vi "CalibrationPathConstants.vi"() -> (0 "PSU3 TachPath":T1=path "Z:/Data/Calibration/Tachometer/PSU3_TachCalibration.csv", 1 "PSU2 RevTachPath":T1=path "Z:/Data/Calibration/Reverse Tachometer/PSU2_RevTachCalibration.csv", 2 "PSU2 TachPath":T1=path "Z:/Data/Calibration/Tachometer/PSU2_TachCalibration.csv", 3 "CryoPath":T1=path "Z:/Data/Calibration/Cryo Temp/CryoTemp.csv", 4 "PSU3 RevTachPath":T1=path "Z:/Data/Calibration/Reverse Tachometer/PSU3_RevTachCalibration.csv")   [LabVIEW 2014]
doc: "This VI defines a hardcoded path constant that is used in the init, MDS+ load and restore default settings.\n\nTo change the hardcode, type in the new path and right-click, select data operations, make current value default and save the VI."
uses:
  CryotempCalPath.ctl
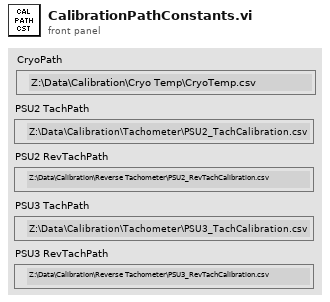
[diagram p1: front panel]
types:
  T1 = typedef "CryotempCalPath.ctl" = path
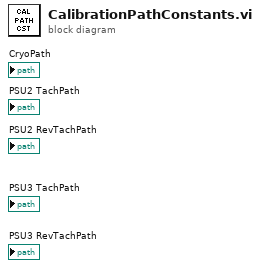
[diagram p0: block diagram]
diagram:
